vi "Module Name--constant.vi"() -> (3 "Module Name":string)   [LabVIEW 2022 SP3, in "MainPanel.lvlib"]
doc: "Return the name of the module that owns this VI. \n_____\nBased on DQMH Project Template 7.0.1.1316."
uses:
  MainPanel.lvlib
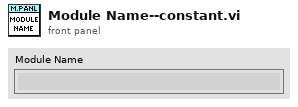
[diagram p1: front panel]
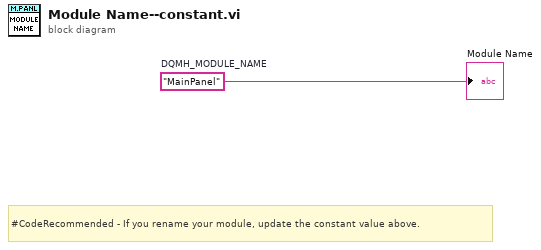
[diagram p0: block diagram]
diagram:
  w1 = "MainPanel"  # DQMH_MODULE_NAME
  # "#CodeRecommended - If you rename your module, update the constant value above."
  "Module Name" <- w1
